vi "Start Stop Integration.vi"(0 "VISA resource name":refnum<visa-resource-name>, 5 "Start/Stop (F: Stop)":bool, 11 "error in (no error)":errorcluster) -> (4 "VISA resource name out":refnum<visa-resource-name>, 15 "error out":errorcluster)   [LabVIEW 2016, in "Yokogawa WT200 Series.lvlib"]
doc: "This VI sends the Integrate start/stop command to the WT200 Series."
uses:
  Yokogawa WT200 Series.lvlib
panel:
  out "output string":string
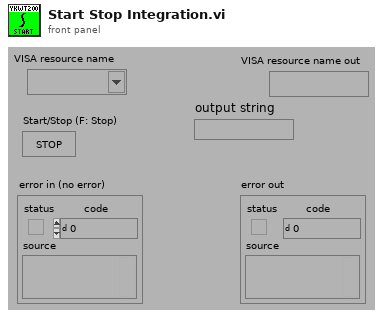
[diagram p1: front panel]
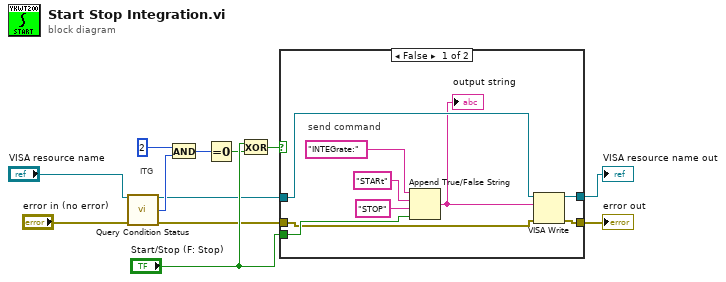
[diagram p0: block diagram]
diagram:
  # "ITG"
  n1 = call "Query Condition Status.vi"("VISA resource name"="VISA resource name", "error in (no error)"="error in (no error)") -> ("VISA resource name out"=w2:refnum<visa-resource-name>, "Condition"=w5:u16, "error out"=w1:errorcluster)  [unwired: 11 in]
  n2 = And(x=u16 2, y=w5) -> (x .and. y?=w9:u16)
  n3 = Equal To 0?(x=w9) -> (x = 0?=w10:bool)
  n4 = Exclusive Or(1:w10, 2:"Start/Stop (F: Stop)") -> (0:w11:bool)
  n5 = case shown="False" w11 {
    tunnel: w1 -> [w17 w23]
    tunnel: [w16 w23] -> w4
    tunnel: "Start/Stop (F: Stop)" -> [w18 _]
    tunnel: w2 -> [w15 w22]
    tunnel: [w14 w22] -> w3
    frame False {
      # "send command"
      n6 = Append True/False String(1:w18, 2:"STOP", 3:"STARt", 4:"INTEGrate:") -> (0:w13:string)
      "output string" <- w13
      n7 = VISA Write(VISA resource name=w15, write buffer=w13, error in (no error)=w17) -> (VISA resource name out=w14:refnum<visa-resource-name>, error out=w16:errorcluster)  [unwired: 1 out]
    }
    frame True {
      # "no change"
    }
  }
  "error out" <- w4
  "VISA resource name out" <- w3
